vi "Main.vi"(8 "error in":errorcluster, 11 "Main UI in":refnum<class "Main UI.lvclass">) -> (0 "error out":errorcluster, 3 "Main UI out":refnum<class "Main UI.lvclass">)   [LabVIEW 2017, in "Main UI.lvclass"]
doc: "The <b>Queued Message Handler</b> of the Worker that owns this VI."
uses:
  Main UI.lvclass
  Client Data.ctl
  Initialization Data.ctl
  Response Cases.ctl
  <vilib>/addons/_Workers/Library/Case Label.ctl
  Main UI.lvclass/Main UI.ctl
  rsp_TCP Server Start Listening.ctl
  rql_Start Exiting Application.ctl
  rqp_TCP Client Connection Notify.ctl
  rqp_TCP Client Incoming Data.ctl
  Shared/Raw FPGA Data.ctl
  rqp_Embed System Monitor UI.ctl
  <vilib>/addons/_Workers/Library/Workers.lvlib
panel:
  in  "Tab Control":T1(tab)
  out "Waveform Chart":cluster{dbl, dbl}[](graph)
  in  "Server Name":string="Host NI 9205 Demo"
  out "Listening":bool
  in  "Server Port":u16=9123
  in  "Start/Stop Listening":bool caption="Disconnect from Server"
  in  "TCP Client":T2
  # "Server Name"
  # "Server Port"
  # "Client Name :"
  # "IP Address :"
  # "Connected? :"
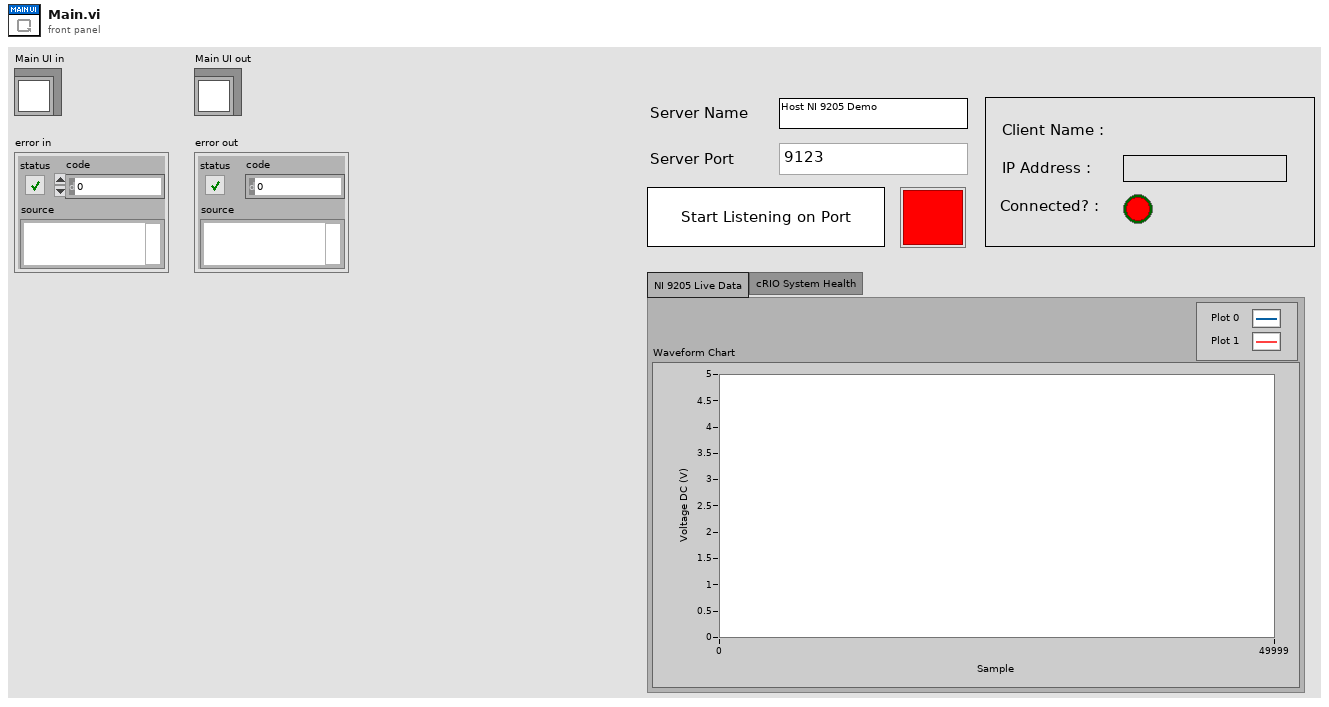
[diagram p1: front panel]
types:
  T1 = enum32{"NI 9205 Live Data", "cRIO System Health"}
  T2 = typedef "Main UI.lvclass/Client Data.ctl" = cluster{"Client Name":string, "IP Address":string, "Connected?":bool}
  T3 = typedef "Main UI.lvclass/Initialization Data.ctl" = cluster{"Response Cases":T4}
  T4 = typedef "Main UI.lvclass/Response Cases.ctl" = cluster{"TCP Server Start Listening":T5, "TCP Server Stop Listening":T5, "Start Exiting Application":T5}
  T5 = typedef "Workers.lvlib/Case Label.ctl" = string
  T6 = typedef "Main UI.lvclass/rsp_TCP Server Start Listening.ctl" = cluster{"Server Name":string, "Server Port":u16}
  T7 = typedef "Main UI.lvclass/rql_Start Exiting Application.ctl" = cluster{"String":string}
  T8 = typedef "Main UI.lvclass/rqp_TCP Client Connection Notify.ctl" = cluster{"Client Name":string, "IP Address":string, "Connected?":bool}
  T9 = typedef "Raw FPGA Data.ctl" = fxp<+/-,26,5>[]
  T10 = typedef "Main UI.lvclass/rqp_TCP Client Incoming Data.ctl" = cluster{"Data as String":string}
  T11 = typedef "Main UI.lvclass/rqp_Embed System Monitor UI.ctl" = cluster{"Main VI Ref":refnum<vi>}
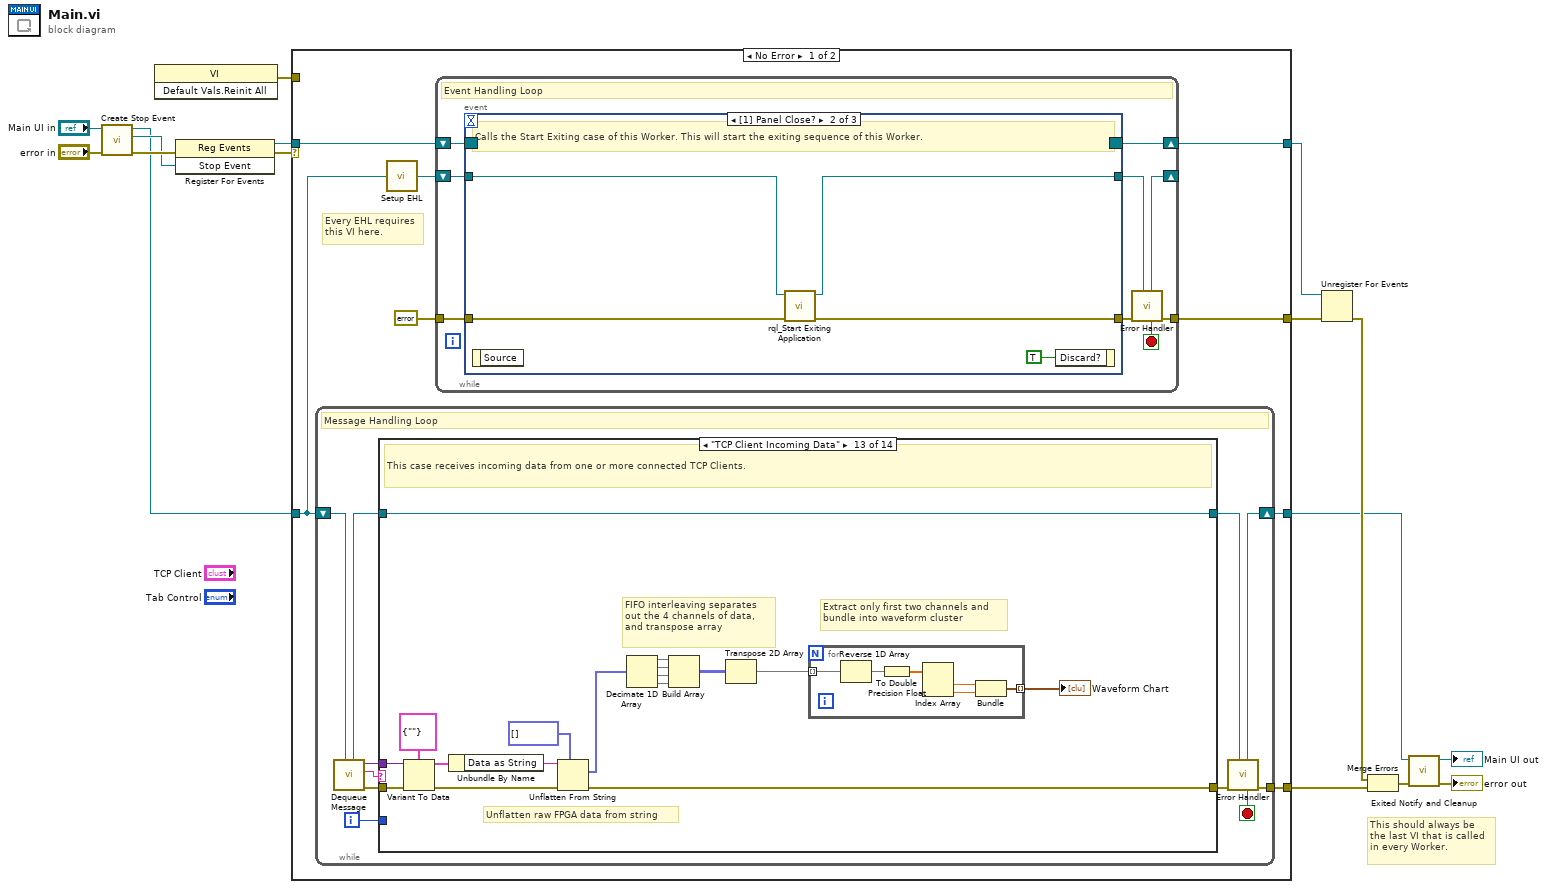
[diagram p0: block diagram]
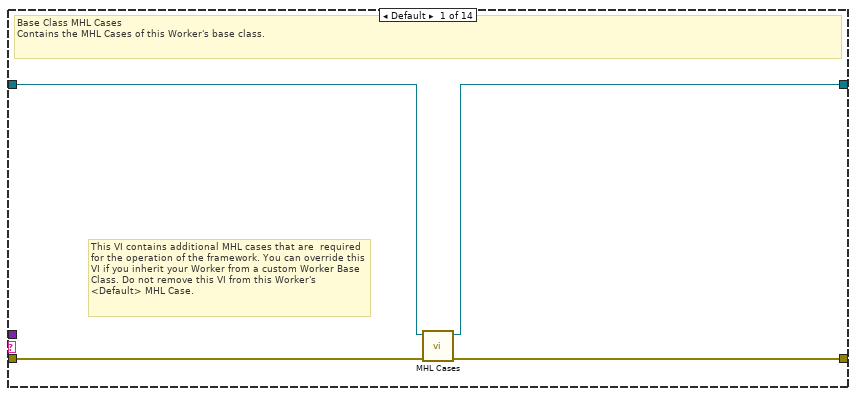
[diagram p2: hidden frame]
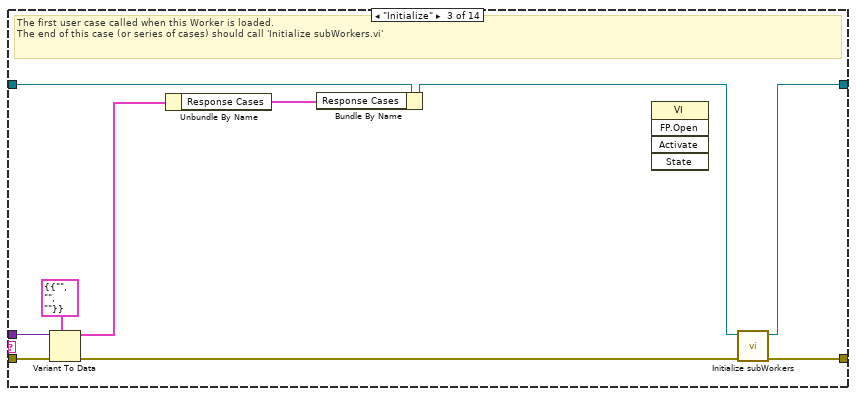
[diagram p4: hidden frame]
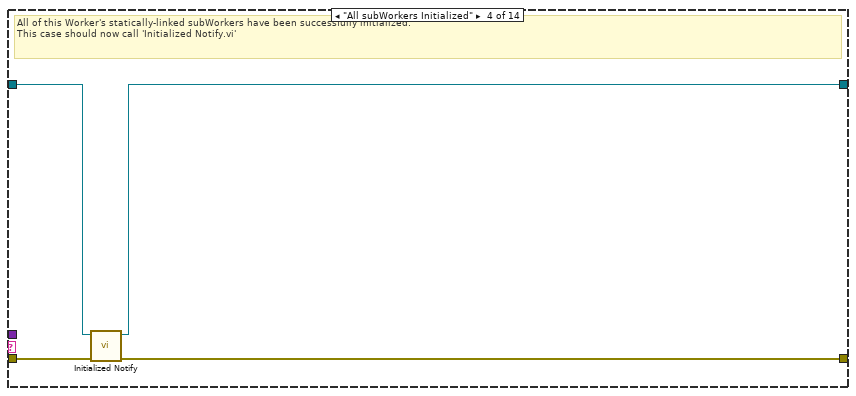
[diagram p5: hidden frame]
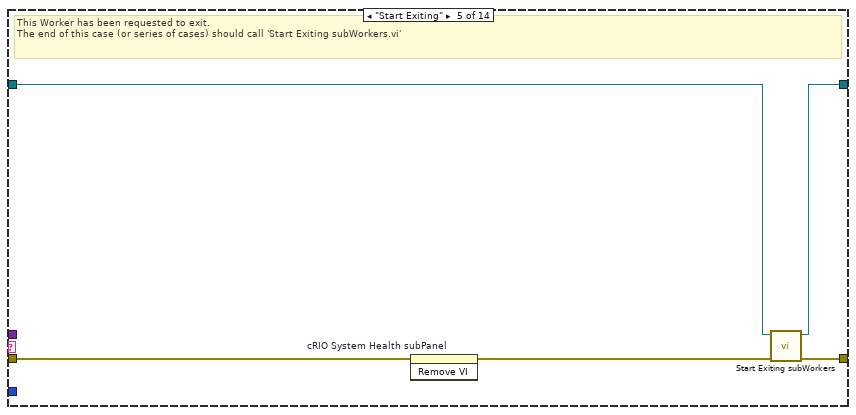
[diagram p6: hidden frame]
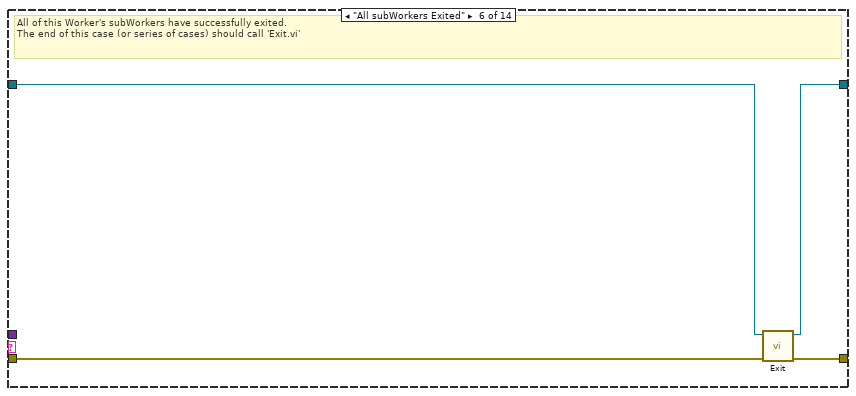
[diagram p7: hidden frame]
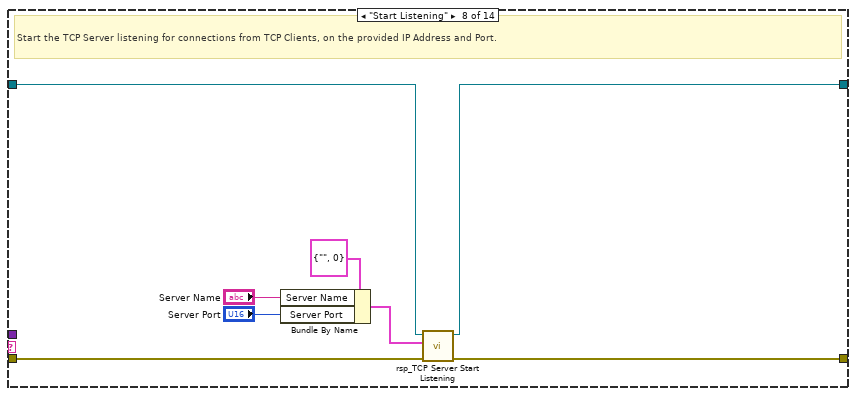
[diagram p9: hidden frame]
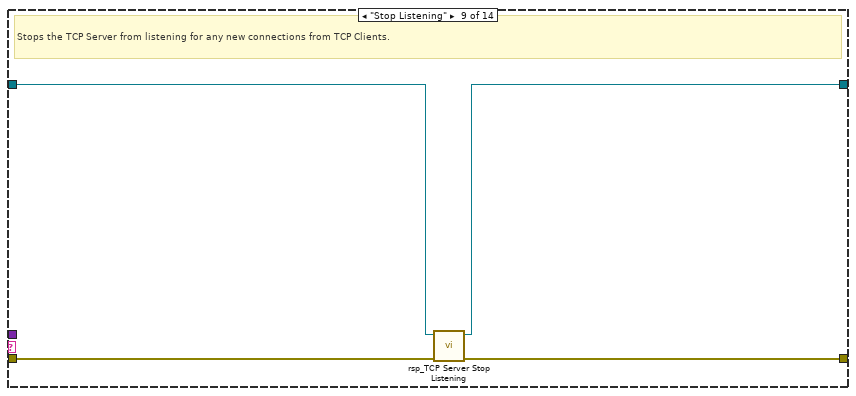
[diagram p10: hidden frame]
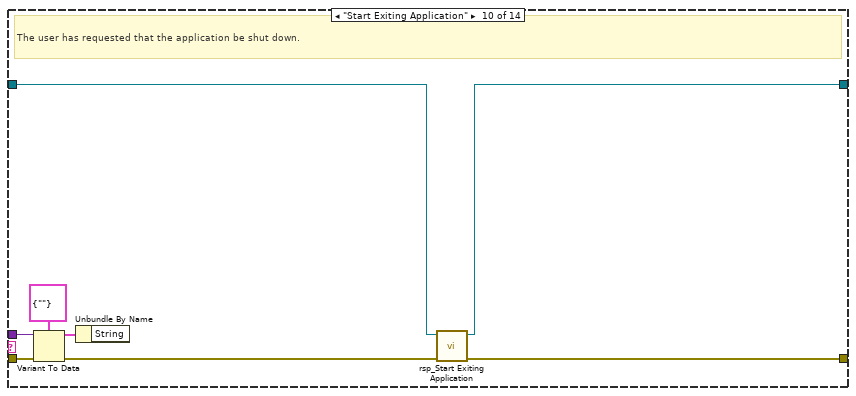
[diagram p11: hidden frame]
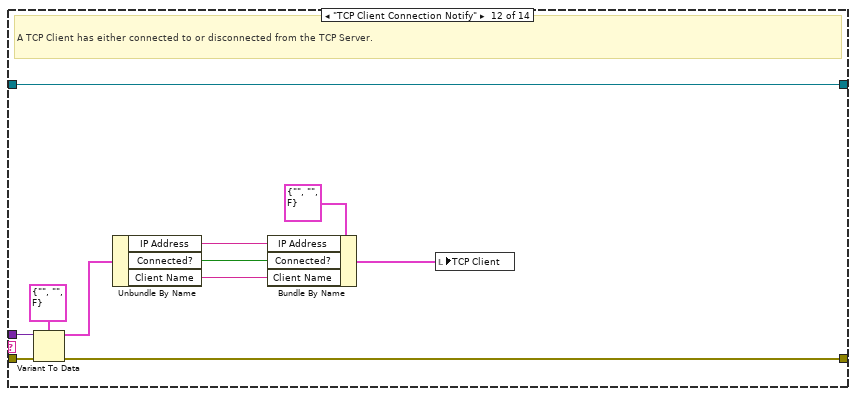
[diagram p13: hidden frame]
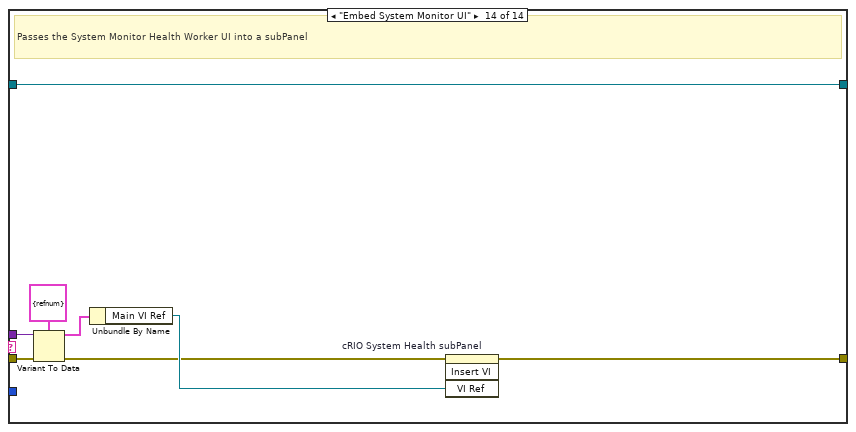
[diagram p14: hidden frame]
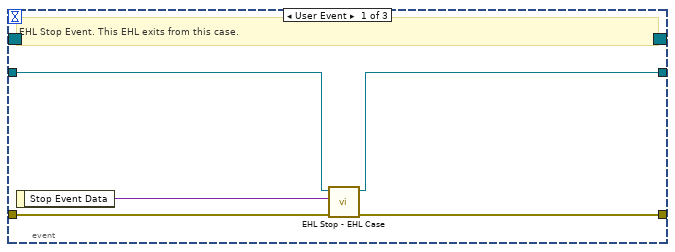
[diagram p15: hidden frame]
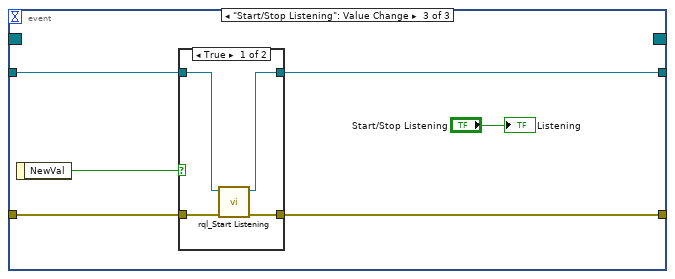
[diagram p16: hidden frame]
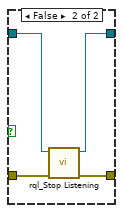
[diagram p17: hidden frame]
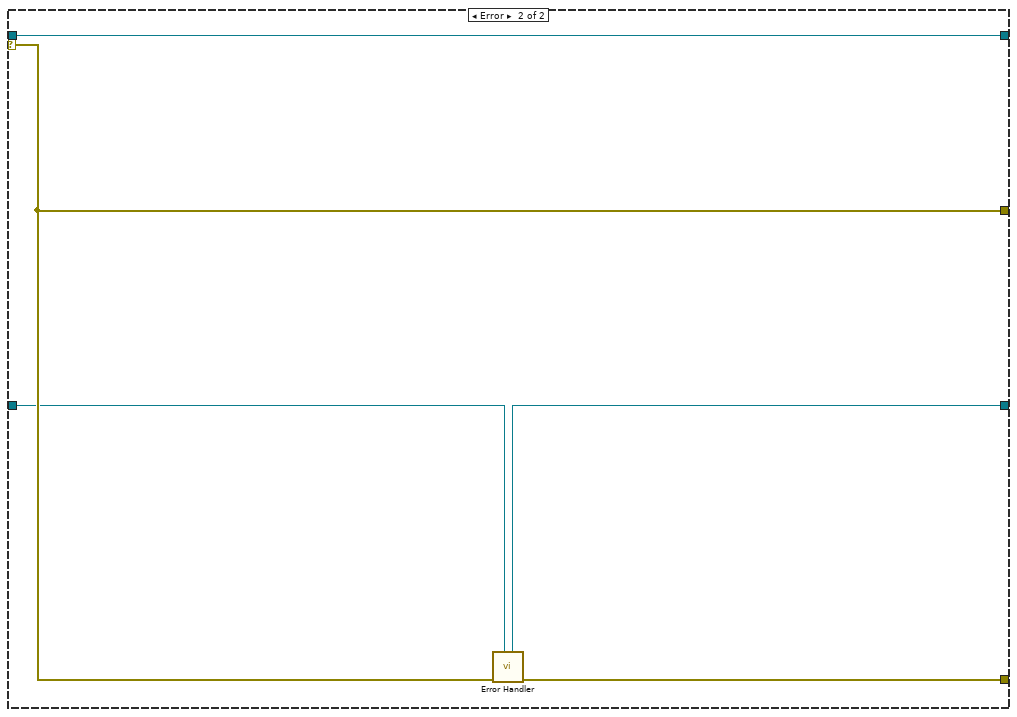
[diagram p18: hidden frame]
diagram:
  # "This should always be the last VI that is called in every Worker."
  n1 = call-dynamic "Create Stop Event.vi"("error in"="error in", "Worker"="Main UI in") -> ("error out"=w11:errorcluster, "Stop Event"=w8:refnum<user-event>, "Worker out"=w5:refnum<class "Main UI.lvclass">)  [unwired: 7 in]
  n2 = invoke class="VI" method="Default Vals.Reinit All"() -> (error out=w3:errorcluster)  [unwired: 3 in, 2 out]
  n3 = register-events(error in=w11, w8) -> (reference out=w10:refnum<event-registration>, error out=w4:errorcluster)  [unwired: 1 in]
  n4 = case shown="No Error" w4 {
    tunnel: w5 -> [w19 w165]
    tunnel: [w17 w166] -> w9
    tunnel: w10 -> [w24 w167]
    tunnel: [w21 w168] -> w15
    tunnel: [w23 w167] -> w14
    tunnel: [w18 w164] -> w12
    selector: w4 -> [_ w168]
    tunnel: w3 -> [_ _]
    frame No Error {
      # "Every EHL requires\nthis VI here."
      n5 = while {
        shift-right: [w33] -> w18
        shift-left: w19 -> [w35]
        tunnel: [w34] -> w17
        i -> [w26]
        stop <- w27 stop-if-true
        # "Message Handling Loop"
        n6 = call-dynamic "Dequeue Message.vi"("Worker"=w35) -> ("error out"=w32:errorcluster, "Case out"=w28:string, "Data out"=w25:variant, "Worker out"=w30:refnum<class "Main UI.lvclass">)  [unwired: 6 in, 1 out]
        n7 = case "Worker MHL Case Structure (DO NOT CHANGE LABEL NAME)" shown="\"TCP Client Incoming Data\"" w28 {
          tunnel: w32 -> [w39 w40 w49 w54 w57 w64 w66 w74 w78 w86 w88 w98 w115 w129]
          tunnel: [w38 w40 w51 w52 w60 w63 w66 w71 w77 w81 w88 w97 w108 w123] -> w31
          tunnel: w30 -> [w37 w41 w45 w55 w58 w62 w65 w69 w75 w80 w87 w99 w116 w130]
          tunnel: [w36 w41 w50 w53 w59 w61 w65 w70 w76 w79 w87 w99 w116 w130] -> w29
          tunnel: w26 -> [_ _ _ _ _ _ _ _ _ _ _ _ _ _]
          tunnel: w25 -> [_ _ w48 _ _ _ _ _ _ w83 _ w95 w113 w127]
          frame Default {
            # "This VI contains additional MHL cases that are  required for the operation of the framework. You can override this VI if you inherit your Worker from a custom Worker Base Class. Do not remove this VI from this Worker's <Default> MHL Case."
            # "Base Class MHL Cases\nContains the MHL Cases of this Worker's base class."
            n8 = call-dynamic "MHL Cases.vi"("error in"=w39, "Worker in"=w37) -> ("error out"=w38:errorcluster, "Worker out"=w36:refnum<class "Main UI.lvclass">)  [unwired: 8 in]
          }
          frame "------------ FRAMEWORK CASES -----------" {
            # "Start of Workers Framework Cases"
          }
          frame "Initialize" {
            # "The first user case called when this Worker is loaded.\nThe end of this case (or series of cases) should call 'Initialize subWorkers.vi'"
            n9 = Variant To Data(error in=w49, type=T3 {"Response Cases"={"TCP Server Start Listening"="", "TCP Server Stop Listening"="", "Start Exiting Application"=""}} ("Initialization Data"), Variant=w48) -> (data=w43:T3, error out=w46:errorcluster)
            n10 = Unbundle By Name(w43) -> ("Response Cases"=w42:T4)
            n11 = Bundle By Name(cluster=w45, "Response Cases"=w42) -> (w44:refnum<class "Main UI.lvclass">)
            n12 = invoke class="VI" method="FP.Open"() -> ()  [unwired: 5 in, 5 out]
            n13 = call-dynamic "Initialize subWorkers.vi"("error in"=w46, "Worker"=w44) -> ("error out"=w51:errorcluster, "dup Worker out"=w50:refnum<class "Main UI.lvclass">)  [unwired: 8 in]
          }
          frame "All subWorkers Initialized" {
            # "All of this Worker's statically-linked subWorkers have been successfully initialized.\nThis case should now call 'Initialized Notify.vi'"
            n14 = call-dynamic "Initialized Notify.vi"("error in"=w54, "Worker"=w55) -> ("error out"=w52:errorcluster, "dup Worker out"=w53:refnum<class "Main UI.lvclass">)  [unwired: 8 in]
          }
          frame "Start Exiting" {
            # "This Worker has been requested to exit. \nThe end of this case (or series of cases) should call 'Start Exiting subWorkers.vi'"
            n15 = invoke on="cRIO System Health subPanel" class="SubPnl" method="Remove VI"(error in=w57) -> (error out=w56:errorcluster)  [unwired: 2 in, 2 out]
            n16 = call-dynamic "Start Exiting subWorkers.vi"("error_in"=w56, "Worker"=w58) -> ("error out"=w60:errorcluster, "dup Worker out"=w59:refnum<class "Main UI.lvclass">)  [unwired: 8 in]
          }
          frame "All subWorkers Exited" {
            # "All of this Worker's subWorkers have successfully exited. \nThe end of this case (or series of cases) should call 'Exit.vi'"
            n17 = call-dynamic "Exit.vi"("error_in"=w64, "Worker"=w62) -> ("error out"=w63:errorcluster, "dup Worker out"=w61:refnum<class "Main UI.lvclass">)  [unwired: 8 in]
          }
          frame "------------- LOCAL API CASES -------------" {
            # "Start of Workers Local API Cases"
          }
          frame "Start Listening" {
            # "Start the TCP Server listening for connections from TCP Clients, on the provided IP Address and Port."
            n18 = Bundle By Name(cluster=T6 {"Server Name"="", "Server Port"=0} ("Data in"), "Server Name"="Server Name", "Server Port"="Server Port") -> (w67:T6)
            n19 = call "rsp_TCP Server Start Listening.vi"("error in"=w74, "Data in"=w67, "Main UI in"=w69) -> ("error out"=w71:errorcluster, "dup Main UI out"=w70:refnum<class "Main UI.lvclass">)  [unwired: 7 in]
          }
          frame "Stop Listening" {
            # "Stops the TCP Server from listening for any new connections from TCP Clients."
            n20 = call "rsp_TCP Server Stop Listening.vi"("error in"=w78, "Main UI in"=w75) -> ("error out"=w77:errorcluster, "dup Main UI out"=w76:refnum<class "Main UI.lvclass">)  [unwired: 8 in]
          }
          frame "Start Exiting Application" {
            # "The user has requested that the application be shut down."
            n21 = Variant To Data(error in=w86, type=T7 {"String"=""} ("Data"), Variant=w83) -> (data=w82:T7, error out=w85:errorcluster)
            n22 = Unbundle By Name(w82) -> ()  [unwired: 1 out]
            n23 = call "rsp_Start Exiting Application.vi"("error in"=w85, "Main UI in"=w80) -> ("error out"=w81:errorcluster, "dup Main UI out"=w79:refnum<class "Main UI.lvclass">)  [unwired: 8 in]
          }
          frame "------------- PUBLIC API CASES -------------" {
            # "Start of Workers Public API Cases"
          }
          frame "TCP Client Connection Notify" {
            # "A TCP Client has either connected to or disconnected from the TCP Server."
            n24 = Variant To Data(error in=w98, type=T8 {"Client Name"="", "IP Address"="", "Connected?"=FALSE} ("Data"), Variant=w95) -> (data=w89:T8, error out=w97:errorcluster)
            n25 = Unbundle By Name(w89) -> ("IP Address"=w93:string, "Connected?"=w94:bool, "Client Name"=w92:string)
            n26 = Bundle By Name(cluster=T2 {"Client Name"="", "IP Address"="", "Connected?"=FALSE} ("Client Connection 1"), "IP Address"=w93, "Connected?"=w94, "Client Name"=w92) -> (w91:T2)
            n27 = local write "TCP Client"(w91) -> ()
          }
          frame "TCP Client Incoming Data" {
            # "Unflatten raw FPGA data from string"
            # "Extract only first two channels and \nbundle into waveform cluster"
            # "FIFO interleaving separates out the 4 channels of data, and transpose array"
            # "This case receives incoming data from one or more connected TCP Clients."
            n28 = Variant To Data(error in=w115, type=T10 {"Data as String"=""} ("Data"), Variant=w113) -> (data=w112:T10, error out=w109:errorcluster)
            n29 = Unbundle By Name(w112) -> ("Data as String"=w110:string)
            n30 = Unflatten From String(type=T9 [] ("Data"), binary string=w110, error in (no error)=w109) -> (value=w103:T9, error out=w108:errorcluster)  [unwired: 2 in, 1 out]
            n31 = Decimate 1D Array(w103) -> (w104:fxp<+/-,26,5>[], w105:fxp<+/-,26,5>[], w106:fxp<+/-,26,5>[], w107:fxp<+/-,26,5>[])
            n32 = Build Array(w104, w105, w106, w107) -> (w101:fxp<+/-,26,5>[][])
            n33 = Transpose 2D Array(2D array=w101) -> (transposed array=w100:fxp<+/-,26,5>[][])
            n34 = for {
              tunnel: w100 -> [w122] mode=indexing
              tunnel: [w119] -> w102 mode=indexing
              n35 = Reverse 1D Array(array=w122) -> (reversed array=w118:fxp<+/-,26,5>[])
              n36 = To Double Precision Float(number=w118) -> (double precision float=w117:dbl[])
              n37 = Index Array(array=w117) -> (element #1=w120:dbl, element #2=w121:dbl)  [unwired: 2 in]
              n38 = Bundle(w120, w121) -> (w119:cluster{dbl, dbl})  [unwired: 1 in]
            }
            "Waveform Chart" <- w102
          }
          frame "Embed System Monitor UI" {
            # "Passes the System Monitor Health Worker UI into a subPanel"
            n39 = Variant To Data(error in=w129, type=T11 {"Main VI Ref"=refnum} ("Data"), Variant=w127) -> (data=w126:T11, error out=w124:errorcluster)
            n40 = Unbundle By Name(w126) -> ("Main VI Ref"=w125:refnum<vi>)
            n41 = invoke on="cRIO System Health subPanel" class="SubPnl" method="Insert VI"(error in=w124, "VI Ref"=w125) -> (error out=w123:errorcluster)  [unwired: 2 in, 3 out]
          }
        }
        n42 = call-dynamic "Error Handler.vi"("Worker"=w29, "error_in"=w31) -> ("error out"=w34:errorcluster, "Stop Loop"=w27:bool, "Worker out"=w33:refnum<class "Main UI.lvclass">)  [unwired: 7 in]
      }
      n43 = call-dynamic "Setup EHL.vi"("Worker"=w19) -> ("Worker out"=w20:refnum<class "Main UI.lvclass">)  [unwired: 14 in]
      n44 = while "Event Handling Loop" {
        shift-right: [w139] -> w23
        shift-left: w24 -> [w138]
        tunnel: [w134] -> w21
        tunnel: errorcluster {"status"=FALSE, "code"=0, "source"=""} ("error constant") -> [w136]
        shift-right: [w132] -> _
        shift-left: w20 -> [w137]
        stop <- w131 stop-if-true
        # "Event Handling Loop"
        n45 = event shown="[1] Panel Close?" {
          selector: w138 -> [_ _ _]
          dyn-events: [_ _ _] -> w139
          timeout: _ -> [_ _ _]
          tunnel: [w143 w148 w153] -> w135
          tunnel: w136 -> [w144 w147 w155]
          tunnel: w137 -> [w142 w145 w152]
          tunnel: [w141 w146 w151] -> w133
          event User Event {
            # "EHL Stop Event. This EHL exits from this case."
            n46 = event-data() -> ("Stop Event Data"=w140:variant)  [unwired: 1 in]
            n47 = call-dynamic "EHL Stop - EHL Case.vi"("error in"=w144, "Stop Event Data"=w140, "Worker"=w142) -> ("error out"=w143:errorcluster, "Worker out"=w141:refnum<class "Main UI.lvclass">)  [unwired: 7 in]
          }
          event Panel Close? {
            # "Calls the Start Exiting case of this Worker. This will start the exiting sequence of this Worker."
            n48 = event-data() -> ()  [unwired: 1 in, 1 out]
            n49 = call "rql_Start Exiting Application.vi"("error in"=w147, "Main UI in"=w145) -> ("error out"=w148:errorcluster, "dup Main UI out"=w146:refnum<class "Main UI.lvclass">)  [unwired: 8 in]
            n50 = event-data ("Event Filter Node")("Discard?"=TRUE) -> ()  [unwired: 1 in, 1 out]
          }
          event "Start/Stop Listening": Value Change {
            n51 = event-data() -> ("NewVal"=w150:bool)  [unwired: 1 in]
            n52 = case shown="True" w150 {
              tunnel: w155 -> [w159 w163]
              tunnel: [w158 w162] -> w153
              tunnel: w152 -> [w157 w161]
              tunnel: [w156 w160] -> w151
              frame True {
                n53 = call "rql_Start Listening.vi"("error in"=w159, "Main UI in"=w157) -> ("error out"=w158:errorcluster, "dup Main UI out"=w156:refnum<class "Main UI.lvclass">)  [unwired: 8 in]
              }
              frame False {
                n54 = call "rql_Stop Listening.vi"("error in"=w163, "Main UI in"=w161) -> ("error out"=w162:errorcluster, "dup Main UI out"=w160:refnum<class "Main UI.lvclass">)  [unwired: 8 in]
              }
            }
            "Listening" <- "Start/Stop Listening"
          }
        }
        n55 = call-dynamic "Error Handler.vi"("Worker"=w133, "error_in"=w135) -> ("error out"=w134:errorcluster, "Stop Loop"=w131:bool, "Worker out"=w132:refnum<class "Main UI.lvclass">)  [unwired: 7 in]
      }
    }
    frame Error {
      n56 = call-dynamic "Error Handler.vi"("Worker"=w165, "error_in"=w168) -> ("error out"=w166:errorcluster, "Worker out"=w164:refnum<class "Main UI.lvclass">)  [unwired: 7 in, 1 out]
    }
  }
  n57 = Unregister For Events(event registration refnum=w14, error in=w15) -> (error out=w16:errorcluster)
  n58 = Merge Errors(w16, w9) -> (w13:errorcluster)
  n59 = call-dynamic "Exited Notify and Cleanup.vi"("error_in"=w13, "Worker"=w12) -> ("error out"=→"error out":errorcluster, "dup Worker out"=→"Main UI out":refnum<class "Main UI.lvclass">)  [unwired: 8 in]
